vi "Write Minimum Size.vi"(5 "Minimum Size":T1, 9 "FPWindow in":refnum<class "FPWindow.lvclass">) -> (3 "FPWindow out":refnum<class "FPWindow.lvclass">)   [LabVIEW 2014, in "Raspberry Pi Compatible Compiler for LabVIEW.lvlib" / "FPWindow.lvclass"]
uses:
  FPWindow.lvclass
  <vilib>/Utility/miscctls.llb/LVPointTypeDef.ctl
  FPWindow.lvclass/FPWindow.ctl
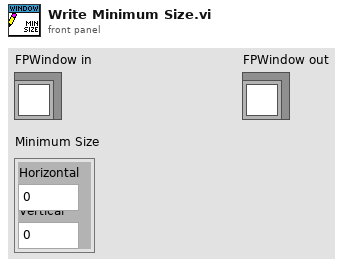
[diagram p1: front panel]
types:
  T1 = typedef "LVPointTypeDef.ctl" = cluster{"Horizontal":i16, "Vertical":i16}
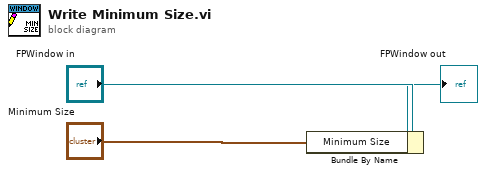
[diagram p0: block diagram]
diagram:
  n1 = Bundle By Name(cluster="FPWindow in", "Minimum Size"="Minimum Size") -> (→"FPWindow out":refnum<class "FPWindow.lvclass">)
